vi "ReadHWState.vi"(8 "error in (no error)":errorcluster, 11 "BME_DG_Base in":refnum<class "BME_DG_Base.lvclass">) -> (0 "error out":errorcluster, 2 "Interrupt Status":u32, 3 "BME_DG_Base out":refnum<class "BME_DG_Base.lvclass">)   [LabVIEW 2009, in "BME_DG_Base.lvclass"]
uses:
  BME_DG_Base.lvclass
  BME_DG_Base.lvclass/BME_DG_Base.ctl
  BME_DG_Chnl/BME_DG_Chnl.lvclass
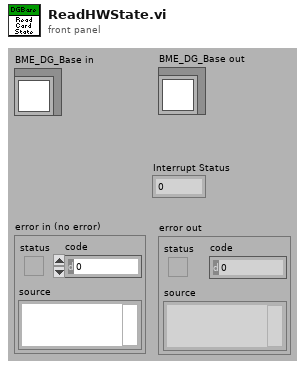
[diagram p1: front panel]
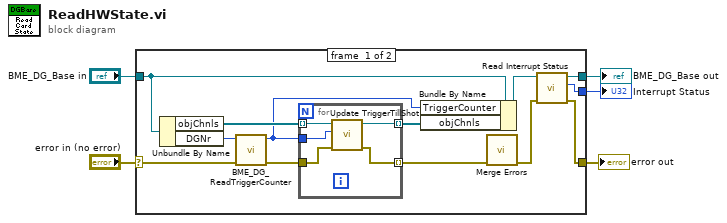
[diagram p0: block diagram]
diagram:
  n1 = case shown="No Error" "error in (no error)" {
    selector: "error in (no error)" -> [w13 w25]
    tunnel: [w9 w25] -> w4
    tunnel: [w11 w24] -> w2
    tunnel: "BME_DG_Base in" -> [w18 w24]
    tunnel: [w8 _] -> w1
    frame #0 {
      n2 = Unbundle By Name(w18) -> ("objChnls"=w16:refnum<class "BME_DG_Chnl.lvclass">[], "DGNr"=w17:i32)
      n3 = call "BME_DG_ReadTriggerCounter.vi"("error in (no error)"=w13, "DG_Number"=w17) -> ("error out"=w15:errorcluster, "return value"=w6:i32)  [unwired: 8 in]
      n4 = for {
        tunnel: w16 -> [w23] mode=indexing
        tunnel: w6 -> [w22]
        tunnel: [w21] -> w14 mode=indexing
        tunnel: w15 -> [w20]
        tunnel: [w19] -> w10 mode=indexing
        n5 = call-dynamic "Update TriggerTillShot.vi"("error in (no error)"=w20, "TriggerCounter"=w22, "BME_DG_Chnl in"=w23) -> ("error out"=w19:errorcluster, "BME_DG_Chnl out"=w21:refnum<class "BME_DG_Chnl.lvclass">)  [unwired: 5 in, 2 out]
      }
      n6 = Bundle By Name(cluster=w18, "TriggerCounter"=w6, "objChnls"=w14) -> (w12:refnum<class "BME_DG_Base.lvclass">)
      n7 = call <vilib>:"Merge Errors.vi"("error array in"=w10) -> ("error out"=w7:errorcluster)  [unwired: 6 in]
      n8 = call-dynamic "Read Interrupt Status.vi"("error in (no error)"=w7, "BME_DG_Base in"=w12) -> ("error out"=w9:errorcluster, "Interrupt Status"=w8:u32, "BME_DG_Base out"=w11:refnum<class "BME_DG_Base.lvclass">)  [unwired: 7 in]
    }
    frame #1 {
    }
  }
  "error out" <- w4
  "BME_DG_Base out" <- w2
  "Interrupt Status" <- w1
